vi "SortRTTraces.vi"(10 "Array in":waveform(dbl)[](array[waveform])) -> (0 "Array 7":waveform(dbl)[](array[waveform]), 2 "Array 5":waveform(dbl)[](array[waveform]), 3 "Array 6":waveform(dbl)[](array[waveform]), 4 "Array 4":waveform(dbl)[](array[waveform]))   [LabVIEW 2024]
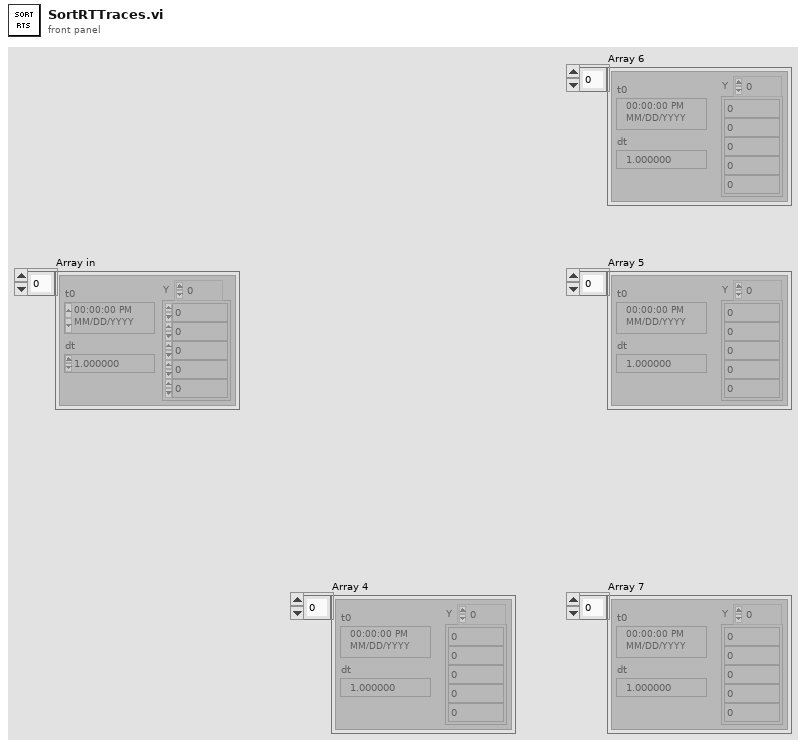
[diagram p1: front panel]
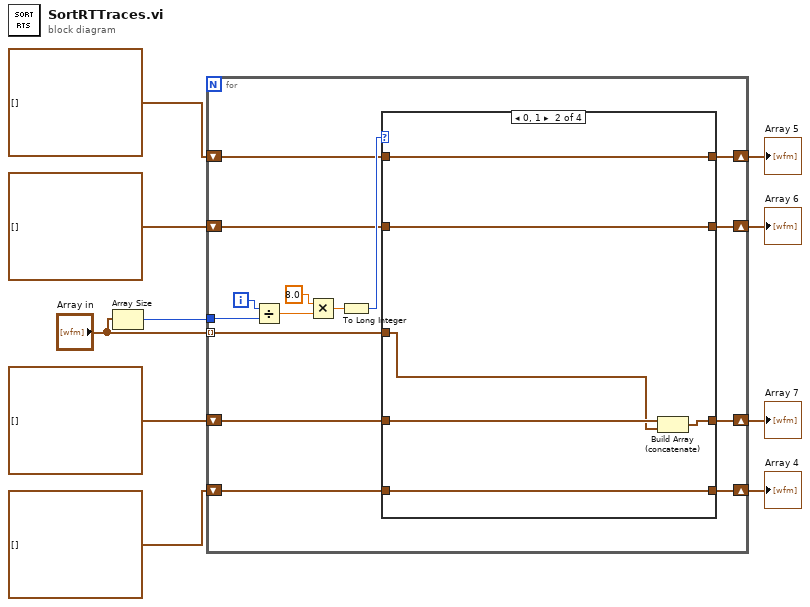
[diagram p0: block diagram]
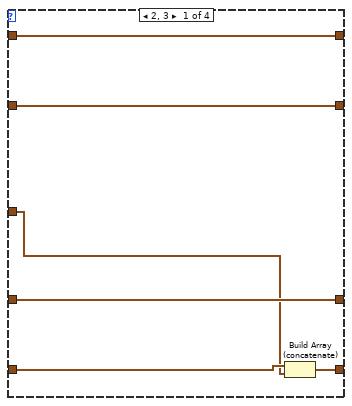
[diagram p2: hidden frame]
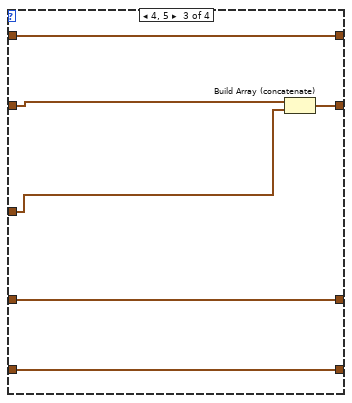
[diagram p3: hidden frame]
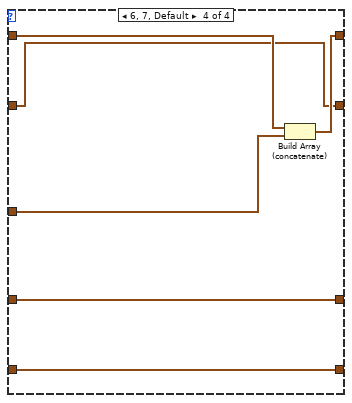
[diagram p4: hidden frame]
diagram:
  n1 = Array Size(array="Array in") -> (size(s)=w5:i32)
  n2 = for {
    tunnel: "Array in" -> [w19] mode=indexing
    shift-right: [w12] -> w10
    shift-left: waveform(dbl)[] [] -> [w11]
    shift-right: [w15] -> w8
    shift-left: waveform(dbl)[] [] -> [w16]
    shift-right: [w14] -> w9
    shift-left: waveform(dbl)[] [] -> [w13]
    shift-right: [w18] -> w7
    shift-left: waveform(dbl)[] [] -> [w17]
    tunnel: w5 -> [w24]
    i -> [w25]
    n3 = Divide(x=w25, y=w24) -> (x/y=w23:dbl)
    n4 = Multiply(x=8.0, y=w23) -> (x*y=w21:dbl)
    n5 = To Long Integer(number=w21) -> (32bit integer=w20:i32)
    n6 = case shown="0, 1" w20 {
      tunnel: w19 -> [w26 w32 w38 w44]
      tunnel: [w29 w37 w41 w47] -> w18
      tunnel: w17 -> [w29 w36 w41 w47]
      tunnel: w16 -> [w28 w35 w43 w46]
      tunnel: [w28 w35 w42 w46] -> w15
      tunnel: [w27 w34 w40 w49] -> w14
      tunnel: w13 -> [w27 w34 w40 w48]
      tunnel: [w31 w33 w39 w45] -> w12
      tunnel: w11 -> [w30 w33 w39 w45]
      frame 2, 3 {
        n7 = Build Array (concatenate)(w30, w26) -> (w31:waveform(dbl)[])
      }
      frame 0, 1 {
        n8 = Build Array (concatenate)(w36, w32) -> (w37:waveform(dbl)[])
      }
      frame 4, 5 {
        n9 = Build Array (concatenate)(w43, w38) -> (w42:waveform(dbl)[])
      }
      frame 6, 7, Default {
        n10 = Build Array (concatenate)(w48, w44) -> (w49:waveform(dbl)[])
      }
    }
  }
  "Array 4" <- w10
  "Array 5" <- w9
  "Array 6" <- w8
  "Array 7" <- w7
